vi "Control Type.vi"(11 "Valve in":refnum<class "LimitControl.lvclass">) -> (2 "Valve Type":string)   [LabVIEW 2020, in "VolatusControl.lvlib" / "LimitControl.lvclass"]
uses:
  LimitControl.lvclass
  LimitControl.lvclass/LimitControl.ctl
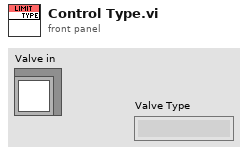
[diagram p1: front panel]
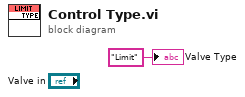
[diagram p0: block diagram]
diagram:
  "Valve Type" <- "Limit" ("Valve Type")
